vi "Write numOfInterleaves.vi"(8 "error in (no error)":errorcluster, 10 "numOfInterleaves":u8, 11 "BuckBoost configuration in":refnum<class "BuckBoost configuration.lvclass">) -> (0 "error out":errorcluster, 3 "BuckBoost configuration out":refnum<class "BuckBoost configuration.lvclass">)   [LabVIEW 2017, in "BuckBoost configuration.lvclass"]
uses:
  BuckBoost configuration.lvclass
  BuckBoost configuration.lvclass/BuckBoost configuration.ctl
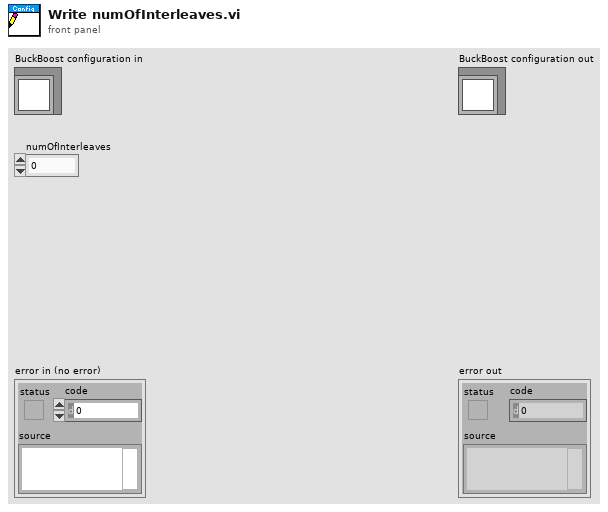
[diagram p1: front panel]
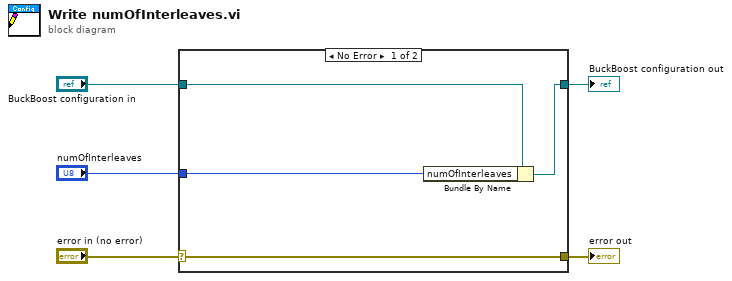
[diagram p0: block diagram]
diagram:
  n1 = case shown="No Error" "error in (no error)" {
    selector: "error in (no error)" -> [w9 w10]
    tunnel: [w9 w10] -> w4
    tunnel: [w7 w11] -> w2
    tunnel: "BuckBoost configuration in" -> [w8 w11]
    tunnel: "numOfInterleaves" -> [w6 _]
    frame No Error {
      n2 = Bundle By Name(cluster=w8, "numOfInterleaves"=w6) -> (w7:refnum<class "BuckBoost configuration.lvclass">)
    }
    frame Error {
    }
  }
  "error out" <- w4
  "BuckBoost configuration out" <- w2
